vi "Set EngineData.vi"(8 "error in (no error)":errorcluster, 11 "HW Engine in":refnum<class "HW Engine.lvclass">) -> (0 "error out":errorcluster, 2 "Engine DataSet":string[][](array[string]), 3 "HW Engine out":refnum<class "HW Engine.lvclass">)   [LabVIEW 2025, in "HW Engine.lvlib" / "HW Engine.lvclass"]
uses:
  HW Engine.lvclass
  C:/Users/Public/Documents/Sandia National Labs/TSS Plugin/CEF.lvlibp/Node/CEF_Node.lvclass
  Users/Public/Documents/Sandia National Labs/TSS Plugin/Abstract Engine.lvlibp/Plugin/Abstract/Abstract Engine/Abstract Engine.lvclass
  Users/Public/Documents/Sandia National Labs/TSS Plugin/CEF.lvlibp/Node/ReadChildren.vi
  Users/Public/Documents/Sandia National Labs/TSS Plugin/Abstract Engine.lvlibp/Plugin/Abstract/Abstract Engine/Read Engine Cluster.vi
  Users/Public/Documents/Sandia National Labs/TSS Plugin/CEF.lvlibp/Node/CEF_Node.lvclass
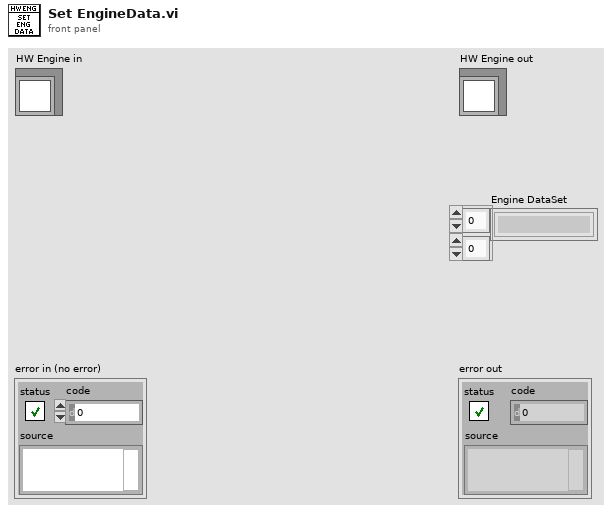
[diagram p1: front panel]
types:
  T1 = typedef "Abstract Engine.lvlibp/Abstract Engine.lvclass/Engine Cluster.ctl" = cluster{"IP Address":string, "Type":string, "Initialized":bool, "InstrumentMap":map{string, cluster{"Initialized":bool, "Channels":T2[]}}}
  T2 = typedef "Abstract Engine.lvlibp/Abstract Instrument.lvclass/Channel.ctl" = cluster{"Alias":string, "Type":enum16{"Numeric", "Boolean", "String"}, "Unit":T3, "Upper limit":dbl, "Lower limit":dbl, "Measurement":variant}
  T3 = typedef "Abstract Engine.lvlibp/Abstract Instrument.lvclass/Unit.ctl" = enum16{"---", "V", "A", "Ohm", "Hz", "uF", "degC", "deg"}
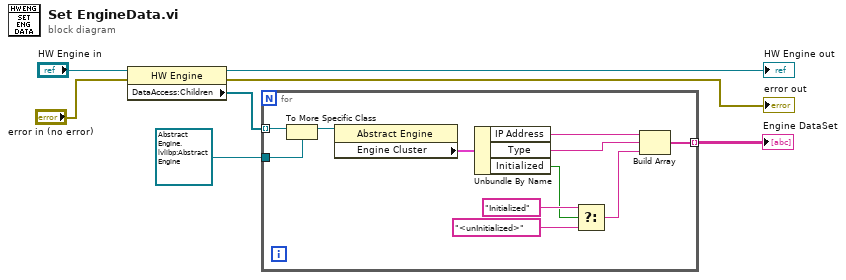
[diagram p0: block diagram]
diagram:
  n1 = property class="HW Engine"(reference="HW Engine in", error in="error in (no error)") -> (reference out=→"HW Engine out":refnum<class "HW Engine.lvclass">, error out=→"error out":errorcluster, "DataAccess:Children"=w5:refnum<data-value>[])
  n2 = for {
    tunnel: w5 -> [w18] mode=indexing
    tunnel: refnum<data-value> refnum ("data value reference") -> [w17]
    tunnel: [w15] -> w3 mode=indexing
    n3 = To More Specific Class(target class=w17, reference=w18) -> (specific class reference=w16:refnum<data-value>)  [unwired: 1 in, 1 out]
    n4 = property class="Abstract Engine"(reference=w16) -> ("Engine Cluster"=w10:T1)  [unwired: 1 in, 2 out]
    n5 = Unbundle By Name(w10) -> ("IP Address"=w9:string, "Type"=w8:string, "Initialized"=w11:bool)
    n6 = Select(t="Initialized" ("Engine"), s=w11, f="<unInitialized>" ("Engine")) -> (s? t:f=w12:string)
    n7 = Build Array(w9, w8, w12) -> (w15:string[])
  }
  "Engine DataSet" <- w3
